vi "Shut Down Hardware.vi"(8 "error in (no error)":errorcluster, 11 "Application in":refnum<class "Application.lvclass">) -> (0 "error out":errorcluster, 3 "Application out":refnum<class "Application.lvclass">)   [LabVIEW 2015]
uses:
  <vilib>/ActorFramework/Stop Msg/Stop Msg.lvclass
  Application.lvclass
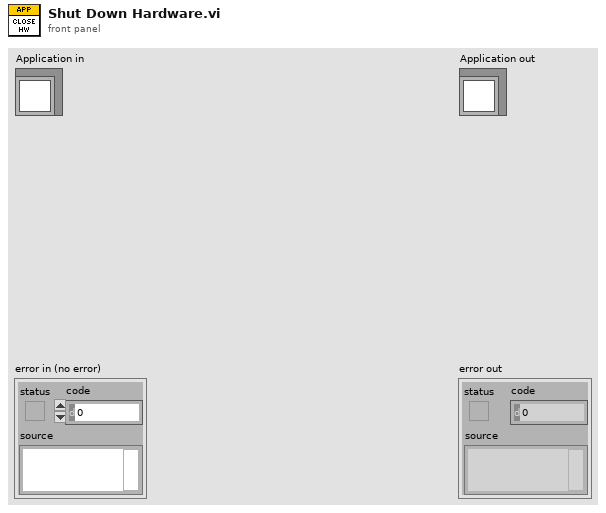
[diagram p1: front panel]
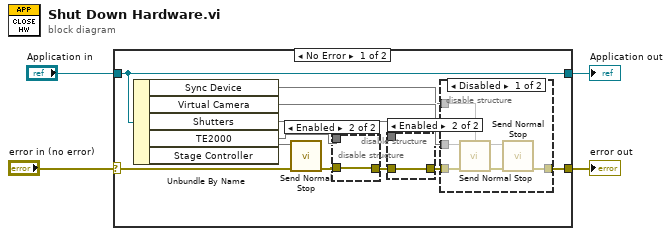
[diagram p0: block diagram]
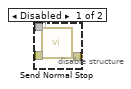
[diagram p2: hidden frame]
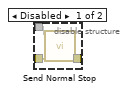
[diagram p3: hidden frame]
diagram:
  n1 = case shown="No Error" "error in (no error)" {
    selector: "error in (no error)" -> [w12 w31]
    tunnel: [w10 w31] -> w3
    tunnel: [w15 w30] -> w1
    tunnel: "Application in" -> [w15 w30]
    frame No Error {
      n2 = Unbundle By Name(w15) -> ("Sync Device"=w5, "Virtual Camera"=w6, "Shutters"=w7, "TE2000"=w8, "Stage Controller"=w9)
      n3 = call <vilib>:"Send Normal Stop.vi"("error in (no error)"=w12, "Message Enqueuer"=w9) -> ("error out"=w11:errorcluster)  [unwired: 9 in]
      n4 = disable-structure shown="Enabled" {
        disable-tunnel: [w18 w19] -> w14
        disable-tunnel: w11 -> [w17 w19]
        disable-tunnel: w8 -> [w16 _]
        frame Disabled {
          n5 = call <vilib>:"Send Normal Stop.vi"("error in (no error)"=w17, "Message Enqueuer"=w16) -> ("error out"=w18:errorcluster)  [unwired: 9 in]
        }
        frame Enabled {
        }
      }
      n6 = disable-structure shown="Enabled" {
        disable-tunnel: w14 -> [w22 w23]
        disable-tunnel: [w21 w23] -> w13
        disable-tunnel: w7 -> [w20 _]
        frame Disabled {
          n7 = call <vilib>:"Send Normal Stop.vi"("error in (no error)"=w22, "Message Enqueuer"=w20) -> ("error out"=w21:errorcluster)  [unwired: 9 in]
        }
        frame Enabled {
        }
      }
      n8 = disable-structure shown="Disabled" {
        disable-tunnel: w13 -> [w28 w29]
        disable-tunnel: [w26 w29] -> w10
        disable-tunnel: w6 -> [w25 _]
        disable-tunnel: w5 -> [w24 _]
        frame Disabled {
          n9 = call <vilib>:"Send Normal Stop.vi"("error in (no error)"=w28, "Message Enqueuer"=w25) -> ("error out"=w27:errorcluster)  [unwired: 9 in]
          n10 = call <vilib>:"Send Normal Stop.vi"("error in (no error)"=w27, "Message Enqueuer"=w24) -> ("error out"=w26:errorcluster)  [unwired: 9 in]
        }
        frame Enabled {
        }
      }
    }
    frame Error {
    }
  }
  "error out" <- w3
  "Application out" <- w1
